vi "S&E Alarm analog String.vi"(2 "Elevated priority":bool, 7 "Content":variant, 9 "error in":errorcluster) -> (8 "format string":string, 10 "error out":errorcluster)   [LabVIEW 2011]
uses:
  reate/S&E Analog Alarm type.ctl
  GUI/Status Indikator Helper.ctl
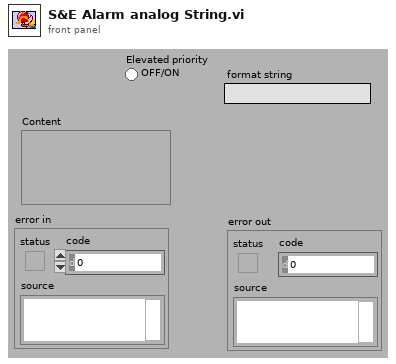
[diagram p1: front panel]
types:
  T1 = typedef "S&E Analog Alarm type.ctl" = cluster{"Alarm":bool, "State":T2, "Value":dbl, "Source name":string}
  T2 = typedef "Status Indikator Helper.ctl" = enum16{"Norm", "L", "H", "LL", "HH", "Value", "Technical"}
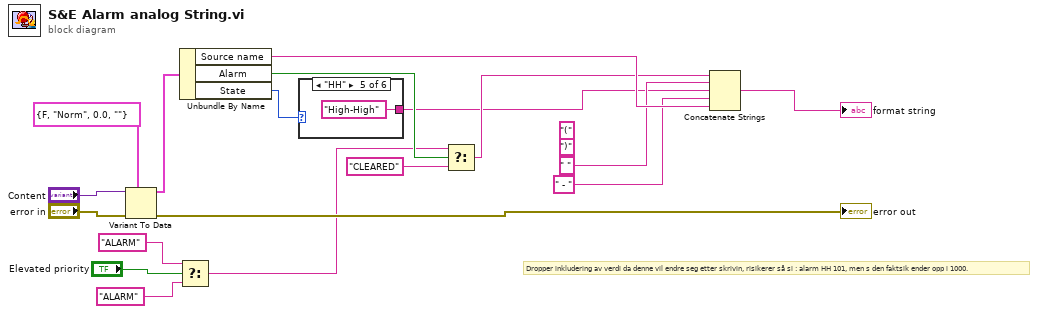
[diagram p0: block diagram]
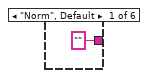
[diagram p2: hidden frame]
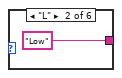
[diagram p3: hidden frame]
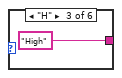
[diagram p4: hidden frame]
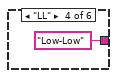
[diagram p5: hidden frame]
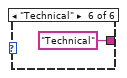
[diagram p6: hidden frame]
diagram:
  (unwired) ")" ("string")
  (unwired) "(" ("string")
  # "Dropper inkludering av verdi da denne vil endre seg etter skrivin, risikerer så si : alarm HH 101, men s den faktsik ender opp i 1000."
  n1 = Variant To Data(error in="error in", type=T1 {"Alarm"=FALSE, "State"=enum."Norm", "Value"=0.0, "Source name"=""} ("S&E Alarm"), Variant="Content") -> (data=w14:T1, error out=→"error out":errorcluster)
  n2 = Unbundle By Name(w14) -> ("Source name"=w9:string, "Alarm"=w8:bool, "State"=w5:T2)
  n3 = Select(t="ALARM" ("string"), s="Elevated priority", f="ALARM") -> (s? t:f=w7:string)
  n4 = case shown="\"HH\"" w5 {
    tunnel: ["" ("string") "Low" ("string") "High" ("string") "Low-Low" ("string") "High-High" ("string") "Technical" ("string")] -> w1
    frame "Norm", Default {
    }
    frame "L" {
    }
    frame "H" {
    }
    frame "LL" {
    }
    frame "HH" {
    }
    frame "Technical" {
    }
  }
  n5 = Select(t=w7, s=w8, f="CLEARED") -> (s? t:f=w3:string)
  n6 = Concatenate Strings(w3, " " ("string"), w1, " - " ("string"), w9) -> (→"format string":string)
